vi "setUp.vi"(8 "error in (no error)":errorcluster, 11 "reference in":refnum<class "SMO.UI_TestCase.lvclass">) -> (0 "error out":errorcluster, 3 "reference out":refnum<class "SMO.UI_TestCase.lvclass">)   [LabVIEW 2013, in "SMO.UI_TestCase.lvclass"]
doc: "setUp runs prior to the test method during test execution. Use this method to initialize any object data required by your tests."
uses:
  SMO.UI_TestCase.lvclass
  src/SMO.UI/SMO.UI.lvclass
  SMO.UI_TestCase.lvclass/SMO.UI_TestCase.ctl
  <vilib>/addons/_JKI Toolkits/VI Tester/TestCase.llb/TestCase.lvclass
  src/SMO/SMO.lvclass
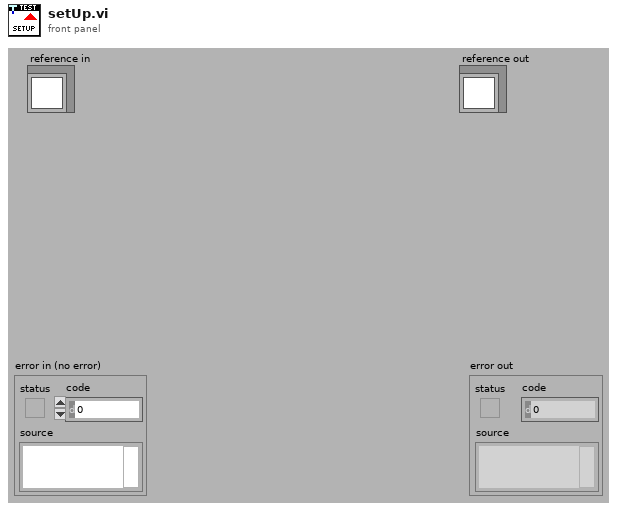
[diagram p1: front panel]
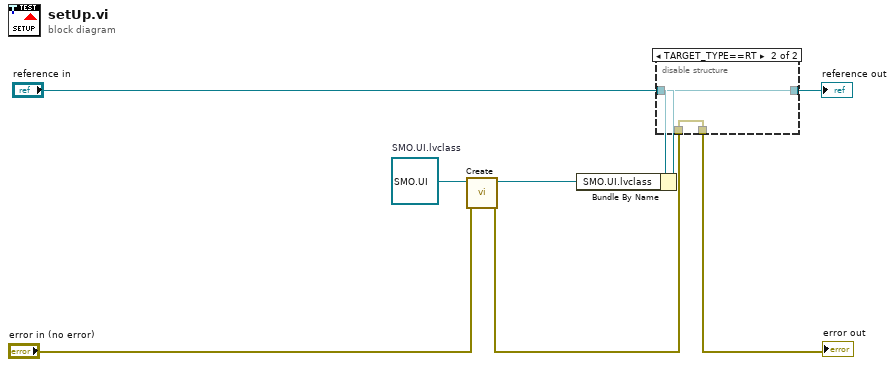
[diagram p0: block diagram]
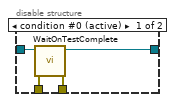
[diagram p2: hidden frame]
diagram:
  w4 = refnum<class "SMO.UI.lvclass"> refnum  # SMO.UI.lvclass
  n1 = call "Create.vi"("error in (no error)"="error in (no error)", "SMO"=w4) -> ("error out"=w1:errorcluster, "SMO out"=w3:refnum<class "SMO.UI.lvclass">)  [unwired: 7 in, 1 out]
  n2 = Bundle By Name(cluster="reference in", "SMO.UI.lvclass"=w3) -> (w5:refnum<class "SMO.UI_TestCase.lvclass">)
  n3 = disable-structure shown="TARGET_TYPE==RT" {
    disable-tunnel: w1 -> [w12 w13]
    disable-tunnel: [w11 w13] -> w8
    disable-tunnel: [w10 w14] -> w6
    disable-tunnel: w5 -> [w9 w14]
    frame condition #0 (active) {
      n4 = call <vilib>:"WaitOnTestComplete.vi"("error in (no error)"=w12, "TestCase in"=w9) -> ("error out"=w11:errorcluster, "TestCase out"=w10:refnum<class "SMO.UI_TestCase.lvclass">)  [unwired: 8 in]
    }
    frame condition #1 {
    }
  }
  "error out" <- w8
  "reference out" <- w6
